vi "CalculateAverageFlux.vi"(8 "Duration":dbl, 9 "Period":dbl, 10 "Flux":dbl, 11 "Total Flux In":dbl) -> (2 "Average Flux":dbl, 3 "Total Flux Out":dbl)   [LabVIEW 2012]
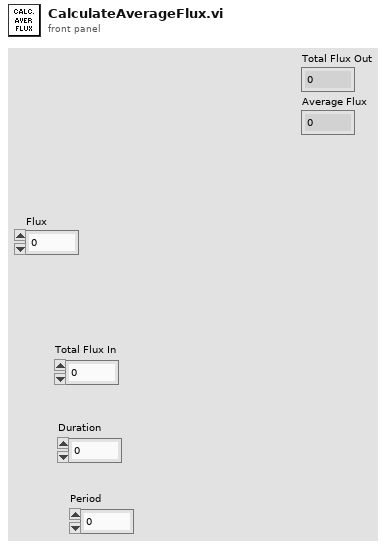
[diagram p1: front panel]
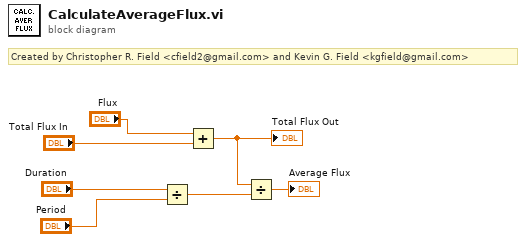
[diagram p0: block diagram]
diagram:
  # "Created by Christopher R. Field <cfield2@gmail.com> and Kevin G. Field <kgfield@gmail.com>"
  n1 = Divide(x="Duration", y="Period") -> (x/y=w2:dbl)
  n2 = Add(x="Flux", y="Total Flux In") -> (x+y=w5:dbl)
  "Total Flux Out" <- w5
  n3 = Divide(x=w5, y=w2) -> (x/y=→"Average Flux":dbl)
